vi "string_split.vi"(7 "char (0x00)":string="\u0000", 11 "data in":string) -> (2 "unterminated?":bool, 3 "messages":string[](array[string]))   [LabVIEW 2017, in "rethinkdb.lvlib"]
uses:
  rethinkdb.lvlib
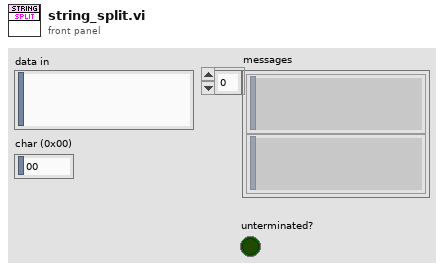
[diagram p1: front panel]
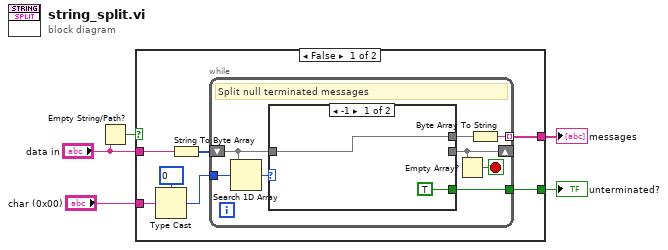
[diagram p0: block diagram]
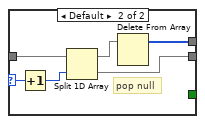
[diagram p2: hidden frame]
diagram:
  n1 = Empty String/Path?(string/path="data in") -> (empty?=w3:bool)
  n2 = case shown="False" w3 {
    tunnel: "data in" -> [w12 _]
    tunnel: [w10 _] -> w5
    tunnel: [w9 _] -> w2
    tunnel: "char (0x00)" -> [w8 _]
    frame False {
      n3 = Type Cast(type=u8 0 ("null"), x=w8) -> (*(type *) &x=w6:u8)
      n4 = String To Byte Array(string=w12) -> (unsigned byte array=w11:u8[])
      n5 = while {
        tunnel: w6 -> [w20]
        shift-right: [w15] -> _
        shift-left: w11 -> [w19]
        tunnel: [w16] -> w10 mode=indexing
        tunnel: [w13] -> w9
        stop <- w14 stop-if-true
        # "Split null terminated messages"
        n6 = Search 1D Array(1D array=w19, element=w20) -> (index of element=w18:i32)  [unwired: 1 in]
        n7 = case shown="-1" w18 {
          selector: w18 -> [_ w27]
          tunnel: w19 -> [w22 w28]
          tunnel: [_ w26] -> w15
          tunnel: [w22 w23] -> w17
          tunnel: [TRUE _] -> w13
          frame -1 {
          }
          frame Default {
            # "pop null"
            n8 = Increment(x=w27) -> (x+1=w25:i32)
            n9 = Split 1D Array(array=w28, index=w25) -> (first subarray=w24:u8[], second subarray=w26:u8[])
            n10 = Delete From Array(array=w24) -> (array with subset deleted=w23:u8[])  [unwired: 2 in, 1 out]
          }
        }
        n11 = Empty Array?(array=w15) -> (empty?=w14:bool)
        n12 = Byte Array To String(unsigned byte array=w17) -> (string=w16:string)
      }
    }
    frame True {
    }
  }
  "unterminated?" <- w2
  "messages" <- w5
